vi "Data Channel Page GUID.vi"() -> (3 "Status GUID":string="6256d297-6817-4828-920b-1215e79da74f")   [LabVIEW 2017, in "DSF Shared.lvlib"]
uses:
  DSF Shared.lvlib
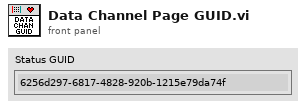
[diagram p1: front panel]
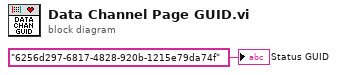
[diagram p0: block diagram]
diagram:
  "Status GUID" <- "6256d297-6817-4828-920b-1215e79da74f" ("Data Sharing Framework")
